vi "mfd_status_text.vi"(8 "Refresh Rate (Hz)":u32=2) -> ()   [LabVIEW 2023]
uses:
  <vilib>/Utility/miscctls.llb/LVBoundsTypeDef.ctl
panel:
  in  "stop":bool
  in  "STATUSTEXT":T1(array[cluster])
  out "MFD_STATUSTEXT":picture
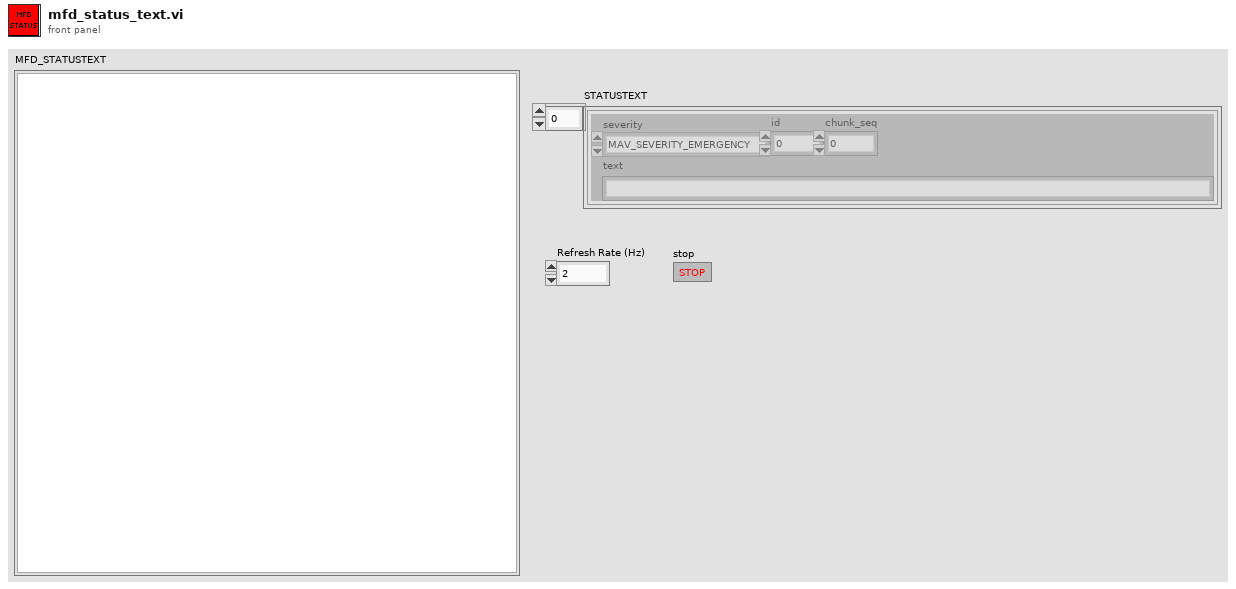
[diagram p1: front panel]
types:
  T1 = cluster{"severity":enum8{"MAV_SEVERITY_EMERGENCY", "MAV_SEVERITY_ALERT", "MAV_SEVERITY_CRITICAL", "MAV_SEVERITY_ERROR", "MAV_SEVERITY_WARNING", "MAV_SEVERITY_NOTICE", "MAV_SEVERITY_INFO", "MAV_SEVERITY_DEBUG"}, "id":u16, "chunk_seq":u8, "text":string}[]
  T2 = cluster{"Font Name:":string, "Size":i16, "Strikeout?":bool, "Italic?":bool, "Underline?":bool, "Outline?":bool, "Shadow?":bool, "Bold?":bool}
  T3 = enum16{"User-specified Font", "Application Font", "System Font", "Dialog Font"}
  T4 = cluster{"horizontal":enum16{"left", "center", "right"}, "vertical":enum16{"top", "center", "bottom"}}
  T5 = cluster{"left":i16, "top":i16, "right":i16, "bottom":i16}
  T6 = cluster{"Width":u16, "Style":enum32{"Solid", "Dash", "Dot", "DashDot", "DashDotDot"}}
  T7 = typedef "LVBoundsTypeDef.ctl" = cluster{"Width":u32, "Height":u32}
  T8 = cluster{"severity":bool, "id":bool, "chunk_seq":bool, "text":bool}[]
  T9 = enum8{"MAV_SEVERITY_EMERGENCY", "MAV_SEVERITY_ALERT", "MAV_SEVERITY_CRITICAL", "MAV_SEVERITY_ERROR", "MAV_SEVERITY_WARNING", "MAV_SEVERITY_NOTICE", "MAV_SEVERITY_INFO", "MAV_SEVERITY_DEBUG"}
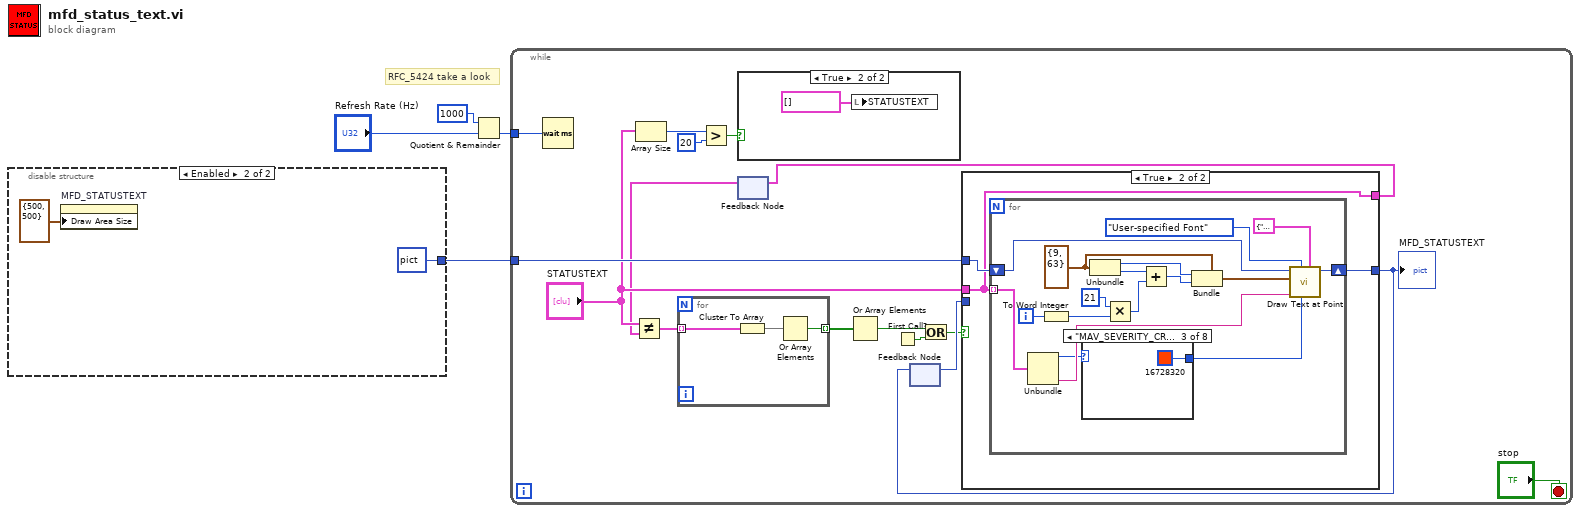
[diagram p0: block diagram]
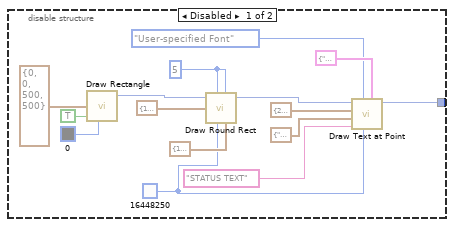
[diagram p2: hidden frame]
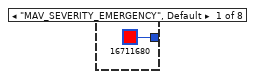
[diagram p4: hidden frame]
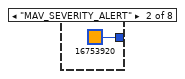
[diagram p5: hidden frame]
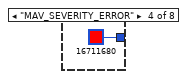
[diagram p6: hidden frame]
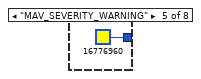
[diagram p7: hidden frame]
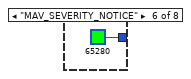
[diagram p8: hidden frame]
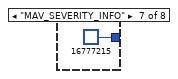
[diagram p9: hidden frame]
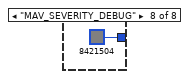
[diagram p10: hidden frame]
diagram:
  # "RFC_5424 take a look"
  n1 = disable-structure shown="Enabled" {
    disable-tunnel: [w5 picture bytes[150] ("new picture")] -> w4
    frame Disabled {
      w12 = u32 16448250 ("text color(black)")
      w15 = i16 5 ("oval height")
      n2 = call <vilib>:"Draw Rectangle.vi"("rect"=T5 {"left"=0, "top"=0, "right"=500, "bottom"=500}, "fill?(F)"=TRUE, "color(black)"=u32 0) -> ("new picture"=w16:picture)  [unwired: 6 in]
      n3 = call <vilib>:"Draw Round Rect.vi"("picture"=w16, "oval width"=w15, "rect"=T5 {"left"=172, "top"=17, "right"=329, "bottom"=47} ("rect 2"), "color(black)"=w12, "oval height"=w15, "pen"=T6 {"Width"=1, "Style"=enum."Solid"}) -> ("new picture"=w6:picture)  [unwired: 3 in]
      n4 = call <vilib>:"Draw Text at Point.vi"("[user-specified font]"=T2 {"Font Name:"="r", "Size"=25, "Strikeout?"=FALSE, "Italic?"=FALSE, "Underline?"=FALSE, "Outline?"=FALSE, "Shadow?"=FALSE, "Bold?"=TRUE}, "text color(black)"=w12, "desired font(Application)"=T3."User-specified Font", "text"="STATUS TEXT", "alignment(left, top)"=T4 {"horizontal"=enum."center", "vertical"=enum."top"}, "origin"=cluster{"x":i16, "y":i16} {"x"=250, "y"=20}, "picture"=w6) -> ("new picture"=w5:picture)  [unwired: 3 in, 1 out]
    }
    frame Enabled {
      n5 = property on="MFD_STATUSTEXT" class="Pict"("Draw Area Size"=T7 {"Width"=500, "Height"=500}) -> ()  [unwired: 2 in, 2 out]
    }
  }
  n6 = Quotient & Remainder(x=u32 1000, y="Refresh Rate (Hz)") -> (floor(x/y)=w1:u32)  [unwired: 1 out]
  n7 = while {
    tunnel: w4 -> [w37]
    tunnel: w1 -> [w23]
    stop <- "stop" stop-if-true
    n8 = Wait (ms)(milliseconds to wait=w23) -> ()  [unwired: 1 out]
    n9 = Array Size(array="STATUSTEXT") -> (size(s)=w36:i32)
    n10 = Greater?(x=w36, y=20) -> (0:w35:bool)
    n11 = case shown="True" w35 {
      frame False {
      }
      frame True {
        n12 = local write "STATUSTEXT"(T1 [] ("STATUSTEXT")) -> ()
      }
    }
    n13 = feedback #1() -> (w31:T1)  [unwired: 1 in]
    n14 = Not Equal?(x="STATUSTEXT", y=w31) -> (x != y?=w28:T8)
    n15 = for {
      tunnel: w28 -> [w40] mode=indexing
      tunnel: [w38] -> w27 mode=indexing
      n16 = Cluster To Array(cluster=w40) -> (array=w39:bool[])
      n17 = Or Array Elements(Boolean array=w39) -> (logical OR=w38:bool)
    }
    n18 = Or Array Elements(Boolean array=w27) -> (logical OR=w26:bool)
    n19 = First Call?() -> (First Call?: T/F=w24:bool)
    n20 = feedback #2() -> (w30:picture)  [unwired: 1 in]
    n21 = Or(x=w26, y=w24) -> (x .or. y?=w25:bool)
    n22 = case shown="True" w25 {
      tunnel: w37 -> [_ w45]
      tunnel: [w41 w44] -> w29
      tunnel: "STATUSTEXT" -> [w42 w43]
      tunnel: [w42 w43] -> w32
      tunnel: w30 -> [w41 _]
      frame False {
      }
      frame True {
        n23 = for {
          tunnel: w43 -> [w46] mode=indexing
          shift-right: [w60] -> w44
          shift-left: w45 -> [w61]
          i -> [w51]
          w59 = cluster{"x":i16, "y":i16} {"x"=9, "y"=63} ("origin")
          n24 = Unbundle(w46) -> ("severity"=w48:T9, "text"=w49:string)  [unwired: 2 out]
          n25 = To Word Integer(number=w51) -> (16bit integer=w50:i16)
          n26 = case shown="\"MAV_SEVERITY_CRITICAL\"" w48 {
            tunnel: [u32 16711680 ("text color(black)") u32 16753920 ("text color(black)") u32 16728320 ("text color(black)") u32 16711680 ("text color(black)") u32 16776960 ("text color(black)") u32 65280 ("text color(black)") u32 16777215 ("text color(black)") u32 8421504 ("text color(black)")] -> w47
            frame "MAV_SEVERITY_EMERGENCY", Default {
            }
            frame "MAV_SEVERITY_ALERT" {
            }
            frame "MAV_SEVERITY_CRITICAL" {
            }
            frame "MAV_SEVERITY_ERROR" {
            }
            frame "MAV_SEVERITY_WARNING" {
            }
            frame "MAV_SEVERITY_NOTICE" {
            }
            frame "MAV_SEVERITY_INFO" {
            }
            frame "MAV_SEVERITY_DEBUG" {
            }
          }
          n27 = Unbundle(w59) -> ("x"=w57:i16, "y"=w52:i16)
          n28 = Multiply(x=i16 21 ("x 2"), y=w50) -> (x*y=w55:i16)
          n29 = Add(x=w52, y=w55) -> (x+y=w56:i16)
          n30 = Bundle(cluster=w59, "x"=w57, "y"=w56) -> (w58:cluster{"x":i16, "y":i16})
          n31 = call <vilib>:"Draw Text at Point.vi"("[user-specified font]"=T2 {"Font Name:"="g", "Size"=20, "Strikeout?"=FALSE, "Italic?"=FALSE, "Underline?"=FALSE, "Outline?"=FALSE, "Shadow?"=FALSE, "Bold?"=TRUE} ("[user-specified font] 2"), "text color(black)"=w47, "desired font(Application)"=T3."User-specified Font", "text"=w49, "origin"=w58, "picture"=w61) -> ("new picture"=w60:picture)  [unwired: 4 in, 1 out]
        }
      }
    }
    "MFD_STATUSTEXT" <- w29
    n32 = feedback-in #1(w32) -> ()
    n33 = feedback-in #2(w29) -> ()
  }
